vi "Instrument.GetPrivateEvents.vi"(8 "error in (no error)":errorcluster, 11 "Instrument":refnum<class "Instrument.lvclass">) -> (0 "error out":errorcluster, 2 "Private Events":T1, 3 "Instrument out":refnum<class "Instrument.lvclass">)   [LabVIEW 2016, in "Instrument.lvclass"]
doc: "---------------------------------------------------------------\nJKI State Machine Objects™\nhttp://jki.net/state-machine-objects/\nCopyright (C) 2005-2015, JKI <info@jki.net>\nALL RIGHTS RESERVEDJKI State Machine Objects (SMO) 1.0.0.4\nJKI - JKI\nCopyright (c) 2015, JKI"
uses:
  Instrument.lvclass
  Typedefs/PrivateEvents--Cluster.ctl
  Typedefs/PrivateEvents--Instrument.SetPort.ctl
  Typedefs/PrivateEvents--Instrument.SetCommands.ctl
  Typedefs/PrivateEvents--Instrument.SetAllowedRemote.ctl
  Instrument.lvclass/Instrument.ctl
panel:
  # "For instructions on how to use the JKI State Machine Objects, examples and video tutorials, visit:\nhttp://jki.net/state-machine-objects/\n\nJKI State Machine Objects™\nhttp://jki.net/state-machine-objects/\nCopyright (C) 2005-2015, JKI <info@jki.net>\nALL RIGHTS RESERVED"
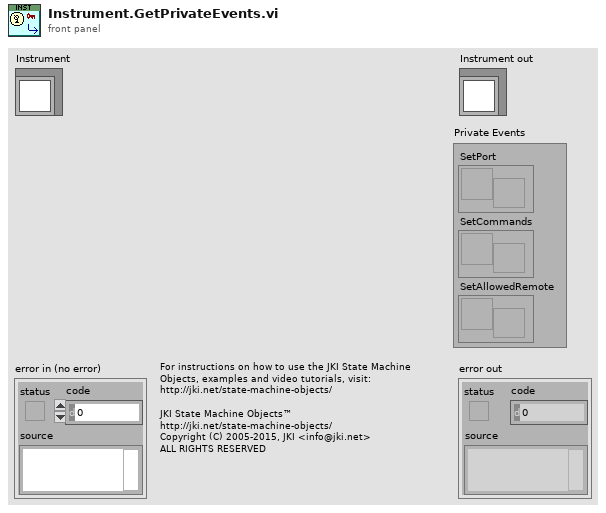
[diagram p1: front panel]
types:
  T1 = typedef "Instrument.lvclass/PrivateEvents--Cluster.ctl" = cluster{"SetPort":refnum<user-event>, "SetCommands":refnum<user-event>, "SetAllowedRemote":refnum<user-event>}
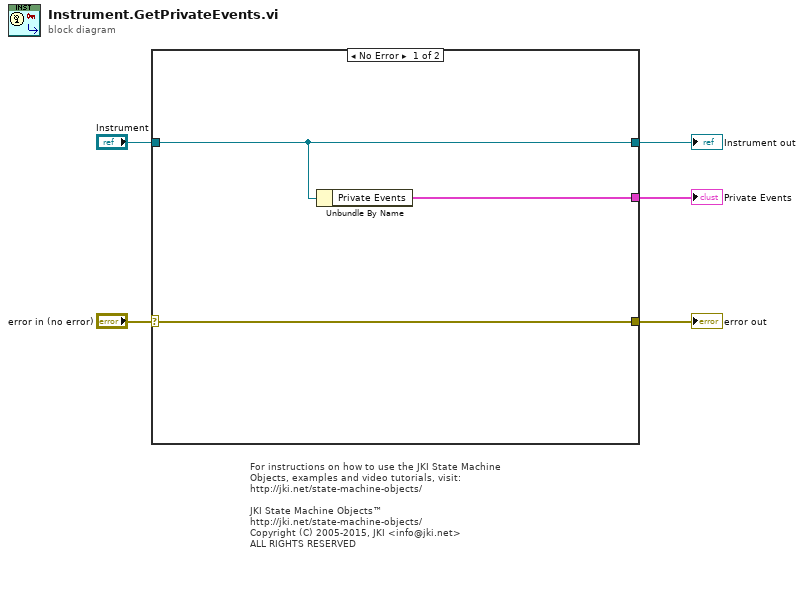
[diagram p0: block diagram]
diagram:
  # "For instructions on how to use the JKI State Machine Objects, examples and video tutorials, visit:\nhttp://jki.net/state-machine-objects/\n\nJKI State Machine Objects™\nhttp://jki.net/state-machine-objects/\nCopyright (C) 2005-2015, JKI <info@jki.net>\nALL RIGHTS RESERVED"
  n1 = case shown="No Error" "error in (no error)" {
    selector: "error in (no error)" -> [w7 w9]
    tunnel: "Instrument" -> [w6 w10]
    tunnel: [w7 w9] -> w4
    tunnel: [w6 w10] -> w3
    tunnel: [w8 _] -> w1
    frame No Error {
      n2 = Unbundle By Name(w6) -> ("Private Events"=w8:T1)
    }
    frame Error {
    }
  }
  "error out" <- w4
  "Instrument out" <- w3
  "Private Events" <- w1
